vi "everest_adc_cap_mismatch.vi"(1 "STG2":dbl, 2 "STG1":dbl, 3 "error in (no error)":errorcluster, 4 "CHB":dbl, 5 "VISA resource name":refnum<visa-resource-name>="COM3") -> (0 "error out":errorcluster)   [LabVIEW 2015]
panel:
  in  "STG1 2":dbl
  in  "STG2 2":dbl
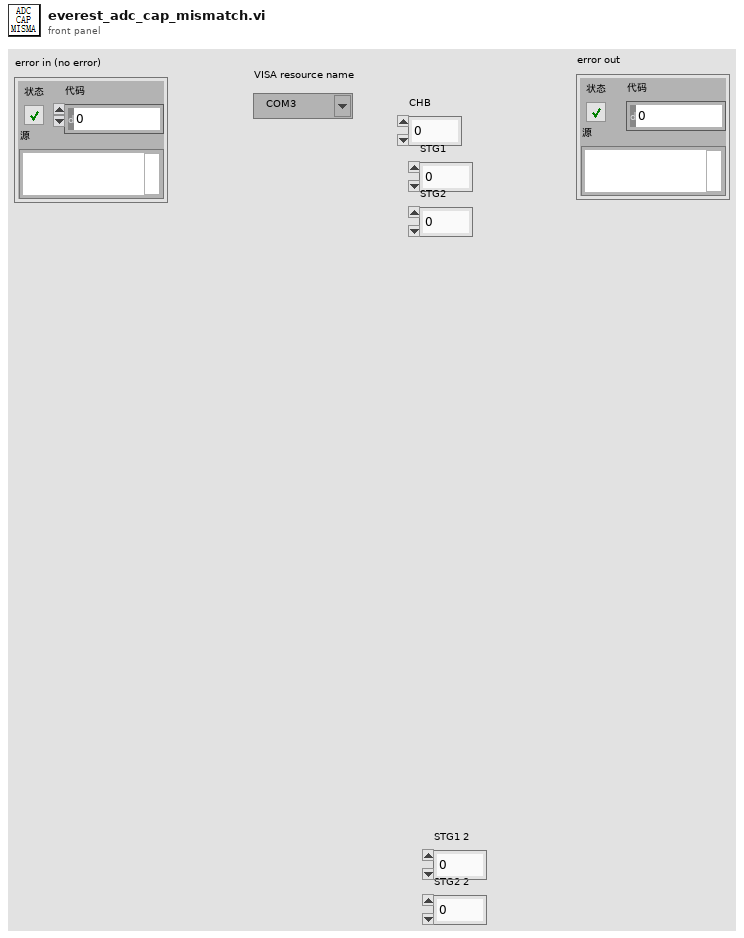
[diagram p1: front panel]
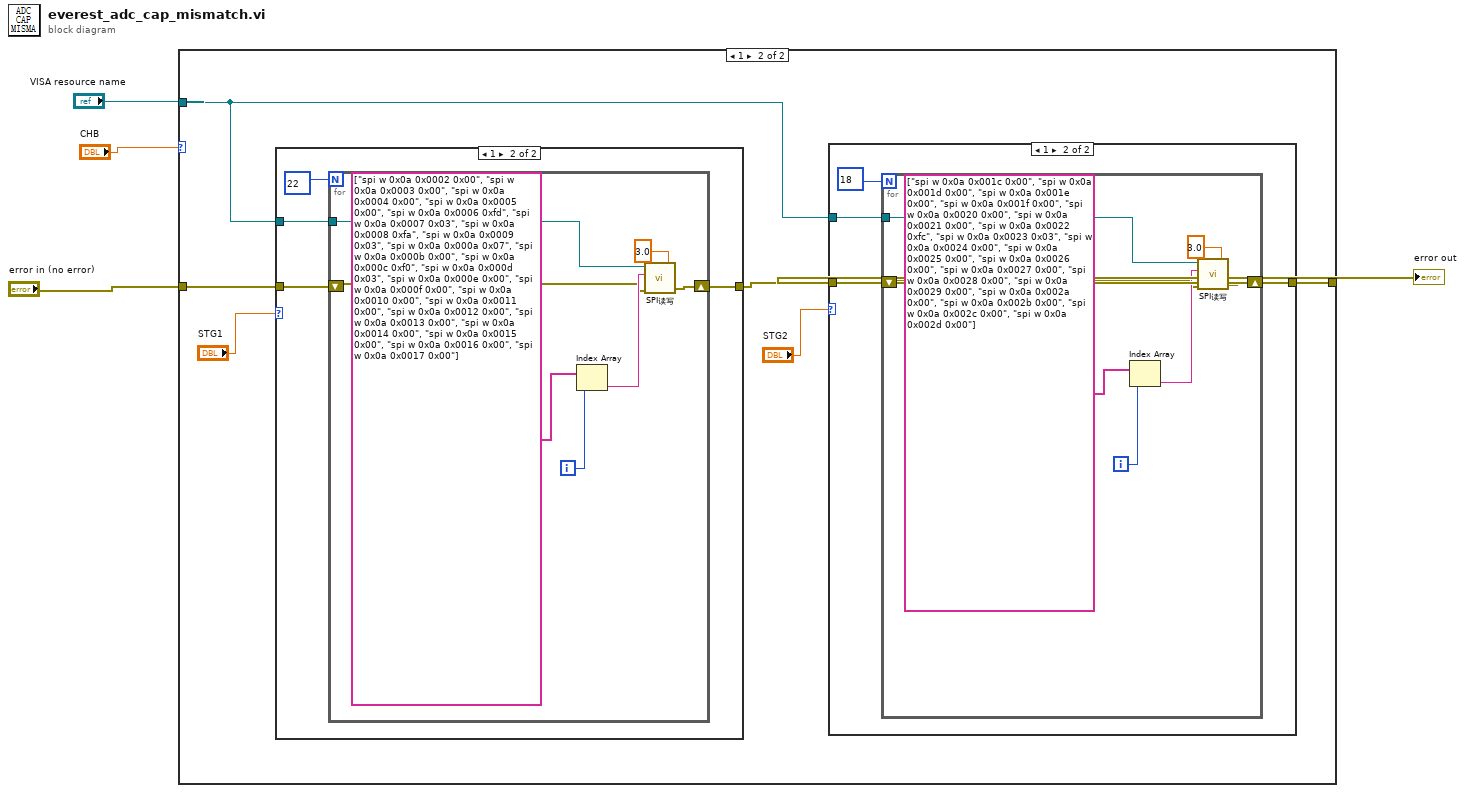
[diagram p0: block diagram]
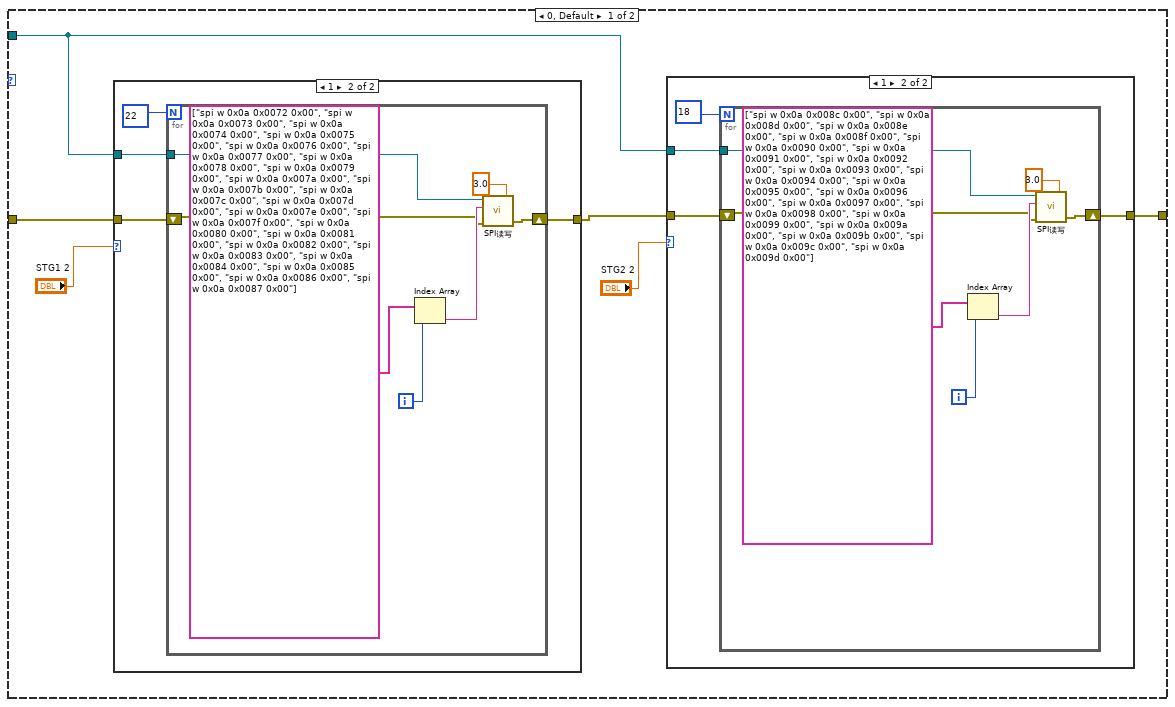
[diagram p2: hidden frame]
diagram:
  n1 = case shown="1" "CHB" {
    tunnel: "error in (no error)" -> [w6 w40]
    tunnel: "VISA resource name" -> [w7 w38]
    tunnel: [w5 w36] -> w3
    frame 0, Default {
      n2 = case shown="1" "STG1 2" {
        tunnel: w6 -> [w23 w27]
        tunnel: w7 -> [_ w26]
        tunnel: [w23 w25] -> w9
        frame 0, Default {
        }
        frame 1 {
          n3 = for {
            N: 22 -> [_]
            tunnel: w26 -> [w30]
            shift-right: [w29] -> w25
            shift-left: w27 -> [w31]
            i -> [w34]
            n4 = Index Array(array=string[] ["spi w 0x0a 0x0072 0x00", "spi w 0x0a 0x0073 0x00", "spi w 0x0a 0x0074 0x00", "spi w 0x0a 0x0075 0x00", "spi w 0x0a 0x0076 0x00", "spi w 0x0a 0x0077 0x00", "spi w 0x0a 0x0078 0x00", "spi w 0x0a 0x0079 0x00", "spi w 0x0a 0x007a 0x00", "spi w 0x0a 0x007b 0x00", "spi w 0x0a 0x007c 0x00", "spi w 0x0a 0x007d 0x00", "spi w 0x0a 0x007e 0x00", "spi w 0x0a 0x007f 0x00", "spi w 0x0a 0x0080 0x00", "spi w 0x0a 0x0081 0x00", "spi w 0x0a 0x0082 0x00", "spi w 0x0a 0x0083 0x00", "spi w 0x0a 0x0084 0x00", "spi w 0x0a 0x0085 0x00", "spi w 0x0a 0x0086 0x00", "spi w 0x0a 0x0087 0x00"], index=w34) -> (element=w32:string)
            n5 = call "SPI读写.vi"("DELAY"=3.0, "error in (no error)"=w31, "往芯片写数据"=w32, "VISA resource name"=w30) -> ("error out"=w29:errorcluster)  [unwired: 1 in, 1 out]
          }
        }
      }
      n6 = case shown="1" "STG2 2" {
        tunnel: w7 -> [_ w15]
        tunnel: [w11 w14] -> w5
        tunnel: w9 -> [w11 w12]
        frame 0, Default {
        }
        frame 1 {
          n7 = for {
            N: 18 -> [_]
            tunnel: w15 -> [w18]
            shift-right: [w17] -> w14
            shift-left: w12 -> [w19]
            i -> [w22]
            n8 = Index Array(array=string[] ["spi w 0x0a 0x008c 0x00", "spi w 0x0a 0x008d 0x00", "spi w 0x0a 0x008e 0x00", "spi w 0x0a 0x008f 0x00", "spi w 0x0a 0x0090 0x00", "spi w 0x0a 0x0091 0x00", "spi w 0x0a 0x0092 0x00", "spi w 0x0a 0x0093 0x00", "spi w 0x0a 0x0094 0x00", "spi w 0x0a 0x0095 0x00", "spi w 0x0a 0x0096 0x00", "spi w 0x0a 0x0097 0x00", "spi w 0x0a 0x0098 0x00", "spi w 0x0a 0x0099 0x00", "spi w 0x0a 0x009a 0x00", "spi w 0x0a 0x009b 0x00", "spi w 0x0a 0x009c 0x00", "spi w 0x0a 0x009d 0x00"], index=w22) -> (element=w20:string)
            n9 = call "SPI读写.vi"("DELAY"=3.0, "error in (no error)"=w19, "往芯片写数据"=w20, "VISA resource name"=w18) -> ("error out"=w17:errorcluster)  [unwired: 1 in, 1 out]
          }
        }
      }
    }
    frame 1 {
      n10 = case shown="1" "STG1" {
        tunnel: w40 -> [w53 w57]
        tunnel: w38 -> [_ w56]
        tunnel: [w53 w55] -> w37
        frame 0, Default {
        }
        frame 1 {
          n11 = for {
            N: 22 -> [_]
            tunnel: w56 -> [w60]
            shift-right: [w59] -> w55
            shift-left: w57 -> [w61]
            i -> [w64]
            n12 = Index Array(array=string[] ["spi w 0x0a 0x0002 0x00", "spi w 0x0a 0x0003 0x00", "spi w 0x0a 0x0004 0x00", "spi w 0x0a 0x0005 0x00", "spi w 0x0a 0x0006 0xfd", "spi w 0x0a 0x0007 0x03", "spi w 0x0a 0x0008 0xfa", "spi w 0x0a 0x0009 0x03", "spi w 0x0a 0x000a 0x07", "spi w 0x0a 0x000b 0x00", "spi w 0x0a 0x000c 0xf0", "spi w 0x0a 0x000d 0x03", "spi w 0x0a 0x000e 0x00", "spi w 0x0a 0x000f 0x00", "spi w 0x0a 0x0010 0x00", "spi w 0x0a 0x0011 0x00", "spi w 0x0a 0x0012 0x00", "spi w 0x0a 0x0013 0x00", "spi w 0x0a 0x0014 0x00", "spi w 0x0a 0x0015 0x00", "spi w 0x0a 0x0016 0x00", "spi w 0x0a 0x0017 0x00"], index=w64) -> (element=w62:string)
            n13 = call "SPI读写.vi"("DELAY"=3.0, "error in (no error)"=w61, "往芯片写数据"=w62, "VISA resource name"=w60) -> ("error out"=w59:errorcluster)  [unwired: 1 in, 1 out]
          }
        }
      }
      n14 = case shown="1" "STG2" {
        tunnel: w38 -> [_ w45]
        tunnel: [w41 w44] -> w36
        tunnel: w37 -> [w41 w42]
        frame 0, Default {
        }
        frame 1 {
          n15 = for {
            N: 18 -> [_]
            tunnel: w45 -> [w48]
            shift-right: [w47] -> w44
            shift-left: w42 -> [w49]
            i -> [w52]
            n16 = Index Array(array=string[] ["spi w 0x0a 0x001c 0x00", "spi w 0x0a 0x001d 0x00", "spi w 0x0a 0x001e 0x00", "spi w 0x0a 0x001f 0x00", "spi w 0x0a 0x0020 0x00", "spi w 0x0a 0x0021 0x00", "spi w 0x0a 0x0022 0xfc", "spi w 0x0a 0x0023 0x03", "spi w 0x0a 0x0024 0x00", "spi w 0x0a 0x0025 0x00", "spi w 0x0a 0x0026 0x00", "spi w 0x0a 0x0027 0x00", "spi w 0x0a 0x0028 0x00", "spi w 0x0a 0x0029 0x00", "spi w 0x0a 0x002a 0x00", "spi w 0x0a 0x002b 0x00", "spi w 0x0a 0x002c 0x00", "spi w 0x0a 0x002d 0x00"], index=w52) -> (element=w50:string)
            n17 = call "SPI读写.vi"("DELAY"=3.0, "error in (no error)"=w49, "往芯片写数据"=w50, "VISA resource name"=w48) -> ("error out"=w47:errorcluster)  [unwired: 1 in, 1 out]
          }
        }
      }
    }
  }
  "error out" <- w3
